vi "QT_ImgSave.vi"(1 "File Settings":T1 {"Dialogs" format="%.0b"}, 2 "Image In":T4 {"Dialogs" format="%.0b"}, 3 "Compression Settings":T3 {"Dialogs" format="%.0b"; "Comp. Quality" format="%.0x"; "Codec" format="%.0x"}, 5 "error in (no error)":errorcluster, 8 "Private":T2) -> (19 "error out":errorcluster)   [LabVIEW 2024]
uses:
  <userlib>/ImageProcessing/QTLIB_2595_LV86/QT_Selector.ctl
  <userlib>/ImageProcessing/QTLIB_2595_LV86/QT_Image.ctl
  <userlib>/ImageProcessing/QTLIB_2595_LV86/QT_Compression.ctl
  <userlib>/ImageProcessing/QTLIB_2595_LV86/QT_Private.ctl
  <userlib>/ImageProcessing/QTLIB_2595_LV86/QT_File.ctl
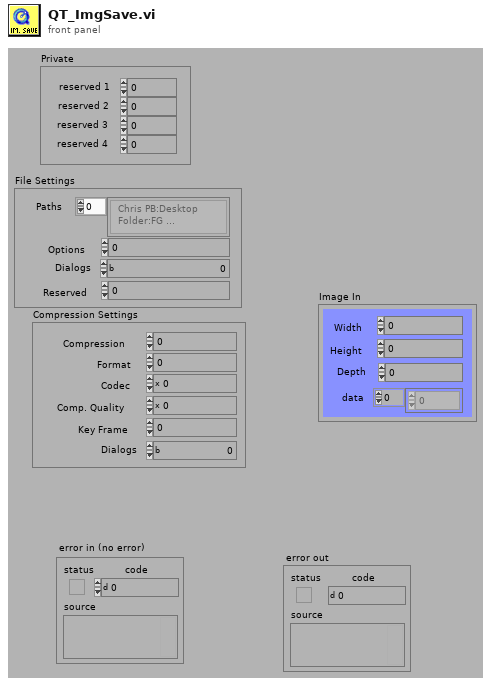
[diagram p1: front panel]
types:
  T1 = typedef "QT_File.ctl" = cluster{"Paths":string[], "Options":i32, "Dialogs":u32, "Reserved":i32}
  T2 = typedef "QT_Private.ctl" = cluster{"reserved 1":i32, "reserved 2":i32, "reserved 3":i32, "reserved 4":i32}
  T3 = typedef "QT_Compression.ctl" = cluster{"Compression":i32, "Format":i32, "Codec":i32, "Comp. Quality":i32, "Key Frame":i32, "Dialogs":u32}
  T4 = typedef "QT_Image.ctl" = cluster{"Width":i32, "Height":i32, "Depth":i32, "data":u8[], "Compressed data":u8[], "Color table":u32[], "Duration":i32, "Options":i32, "Timestamp":i32, "ID":i32, "Reserved":i32, "Dialogs":u32}
  T5 = typedef "QT_Selector.ctl" = enum32{"do nothing", "Get all Sources", "Get Source info", "Open Image", "Save Image to File", "Effect", "Close", "SG Grab", "Compress in Memory", "Decompress to Memory", "New Movie", "Open Movie", "Add Frame", "Get Frame", "Close Movie", "Get QT & CIN info", "SG init", "SG Close", "Open sound file", "Close sound file", "Read sound data", "Write sound data", "Import sound", "Export sound", "Add sound to movie", "Get sound from movie", "reserved", "reserved 1", "reserved 2"}
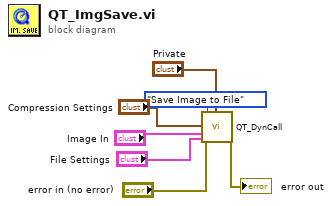
[diagram p0: block diagram]
diagram:
  n1 = call <userlib>:"QT_DynCall.vi"("Compression Settings"="Compression Settings", "Image in"="Image In", "error in (no error)"="error in (no error)", "Selector"=QT_Selector."Save Image to File", "Private"="Private", "File Settings"="File Settings") -> ("error out"=→"error out":errorcluster)  [unwired: 6 in, 15 out]
